vi "Object Tracking V2.vi"() -> ()   [LabVIEW 2019]
uses:
  <vilib>/userdefined/High Color/IMAQdx.ctl
  <vilib>/vision/Pattern Matching.llb/IMAQ Curve Parameters.ctl
  <vilib>/vision/driver/IMAQdx.llb/IMAQdx Buffer Number Mode.ctl
  <vilib>/vision/driver/NI_Vision_Acquisition_Software.lvlib
  <vilib>/vision/NI_Vision_Development_Module.lvlib
  <resource>/objmgr/imaqdx.rc
panel:
  out "Tracking":cluster{"x":dbl, "y":dbl}[](array[cluster])
  in  "Match Type":enum16{"Geometric Matching", "Pattern Matching"}(ring)=enum."Pattern Matching"
  in  "Match":bool
  out "Matches":T1(array[cluster]) {"Bounding Box"."y" format="%.2f"; "Bounding Box"."x" format="%.2f"; "Position"."y" format="%.2f"; "Position"."x" format="%.2f"; "Score" format="%.2f"; "Scale" format="%.2f"; "Angle" format="%.2f"}
  in  "Learn":bool
  in  "Snap Frame":bool
  in  "Camera Name":T2="cam0"
  in  "Stop Button":bool
  in  "Geometric Match Mode":T3={"Rotation"=TRUE, "Scale"=FALSE, "Occlusion"=FALSE, "Reserved"=FALSE, "Reserved"=FALSE, "Reserved"=FALSE}
  in  "Pattern Match Mode":u16(ring)=1 items=["Shift Invariant", "Rotation Invariant"]
  in  "Minimum Score":sgl=600.0
  in  "Nb of Matches":i32=1
  in  "Subpixel Accuracy":bool
  in  "Minimum Contrast":i32=10
  in  "Curve Parameters":T4={"Extraction Mode"=0, "Edge Threshold"=75, "Edge Filter Size"=1, "Min Length"=25, "Row Search Step Size"=15, "Col Search Step Size"=15, "Max Endpoint Gap"=10, "Closed"=FALSE, "Subpixel"=FALSE} {"Max Endpoint Gap" min=0; "Col Search Step Size" min=1 max=255 step=1; "Row Search Step Size" min=1 max=255 step=1; "Min Length" min=0; "Edge Filter Size" items=["Fine", "Normal", "Controur Tracing"]; "Edge Threshold" min=1 max=65535 step=1; "Extraction Mode" items=["Normal", "Uniform Regions"]}
  out "Template":T5(plugin-control)
  out "Snap Image":T5(plugin-control)
  out "Image Out":T5(plugin-control)
  # "1. Run the VI\n\n2. Click \"Snap Frame\" (make sure the object that you want to track\nit in the image at the time you snap the frame\n\n3. Use the mouse to select that object that you wish to track. This is done in the bottow left frame,\n\n4. Click \"Learn\" (This area is not saved at the new template image as seen in the bottom right frame)\n\n5. Click \"Match\" the program will then look for the template image and display the resutls with a red box."
  # "1."
  # "2."
  # "3."
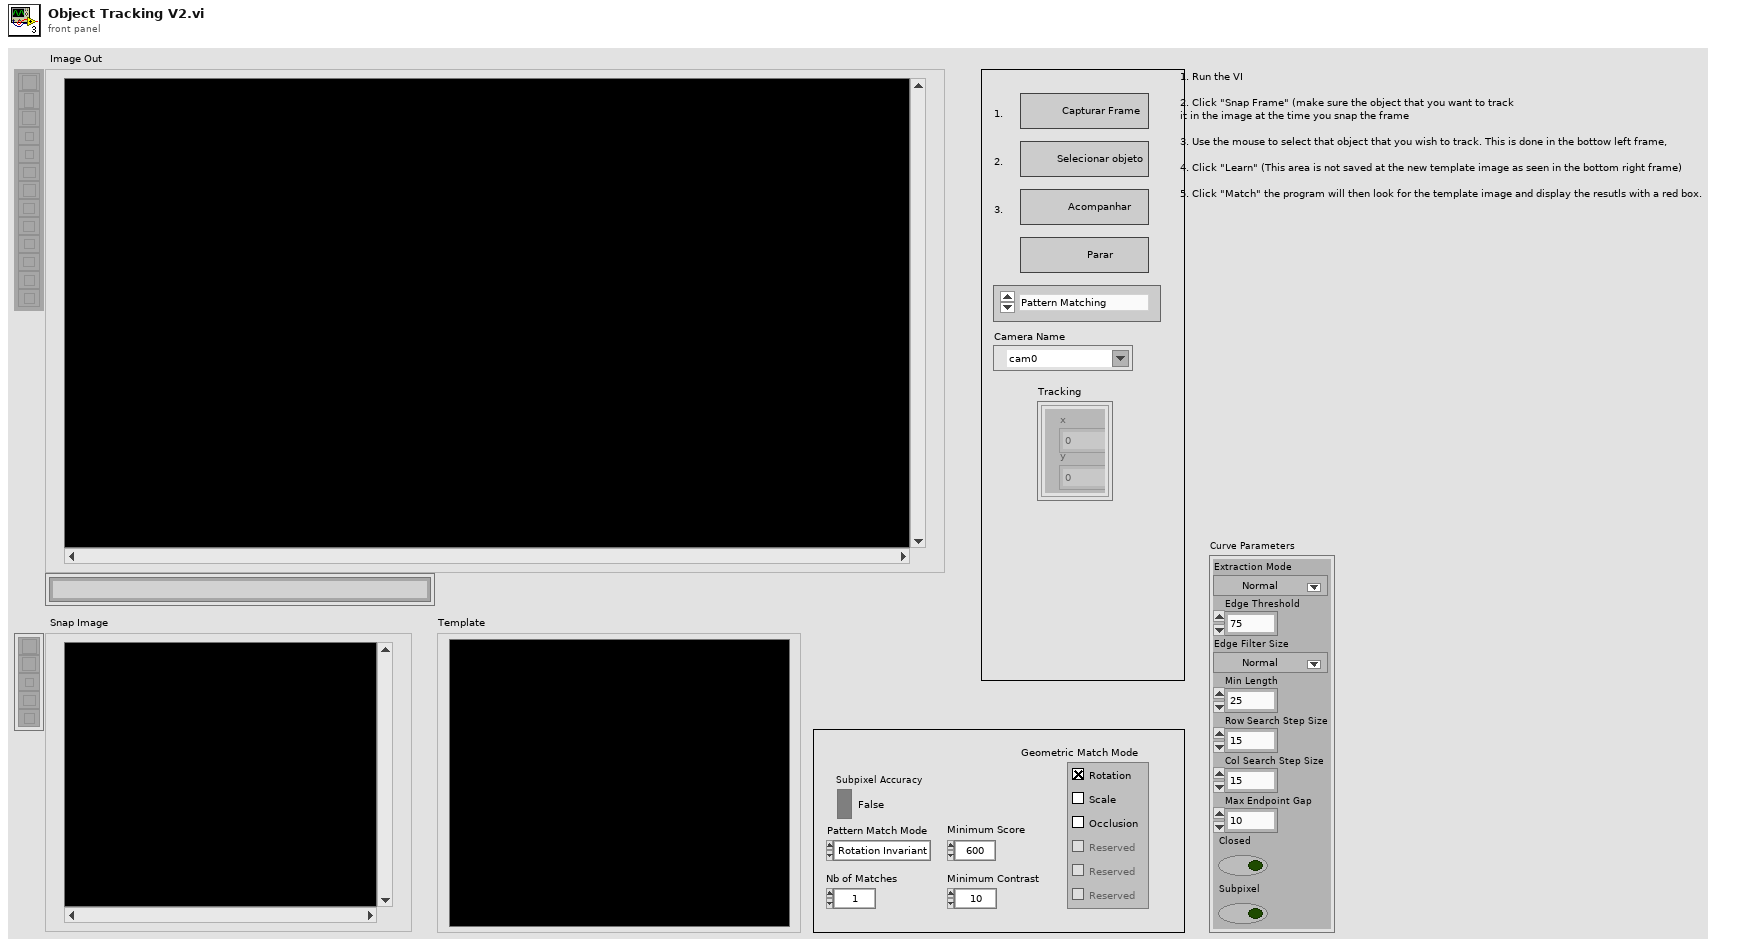
[diagram p1: front panel]
types:
  T1 = cluster{"Position":cluster{"x":sgl, "y":sgl}, "Angle":sgl, "Scale":sgl, "Score":sgl, "Bounding Box":cluster{"x":sgl, "y":sgl}[]}[]
  T2 = typedef "IMAQdx.ctl" = refnum<k21>
  T3 = cluster{"Rotation":bool, "Scale":bool, "Occlusion":bool, "Reserved":bool, "Reserved":bool, "Reserved":bool}
  T4 = typedef "IMAQ Curve Parameters.ctl" = cluster{"Extraction Mode":u32, "Edge Threshold":i32, "Edge Filter Size":u32, "Min Length":i32, "Row Search Step Size":i32, "Col Search Step Size":i32, "Max Endpoint Gap":i32, "Closed":bool, "Subpixel":bool}
  T5 = typedef "IMAQ Image.ctl" = refnum<image>
  T6 = cluster{"Global Rectangle":i32[], "Contours":cluster{"Contour Type":u32, "ROI Type":u32, "Points":i32[]}[]}
  T7 = typedef "NI_Vision_Acquisition_Software.lvlib/IMAQdx Buffer Number Mode.ctl" = enum32{"Next", "Last", "Buffer Number", "Every", "Last New"}
  T8 = cluster{i32[], cluster{"Contour Type":u32, "ROI Type":u32, i32[]}[]}
  T9 = typedef "Image Type" = u32
  T10 = typedef "IMAQ GM Match Report.ctl" = cluster{"Position":cluster{"x":sgl, "y":sgl}, "Angle":sgl, "Scale":sgl, "Score":sgl, "Bounding Box":cluster{"x":sgl, "y":sgl}[], "Contrast Reversed":bool, "Occlusion %":sgl, "Template Target Curve Score":sgl, "Target Template Curve Score":sgl, "Correlation Score":sgl}
  T11 = cluster{"Matches[0]":cluster{"Position":cluster{"x":sgl, "y":sgl}, "Angle":sgl, "Scale":sgl, "Score":sgl, "Bounding Box":cluster{"x":sgl, "y":sgl}[]}, "Matches[1]":cluster{"Position":cluster{"x":sgl, "y":sgl}, "Angle":sgl, "Scale":sgl, "Score":sgl, "Bounding Box":cluster{"x":sgl, "y":sgl}[]}, "Matches[2]":cluster{"Position":cluster{"x":sgl, "y":sgl}, "Angle":sgl, "Scale":sgl, "Score":sgl, "Bounding Box":cluster{"x":sgl, "y":sgl}[]}, "Matches[3]":cluster{"Position":cluster{"x":sgl, "y":sgl}, "Angle":sgl, "Scale":sgl, "Score":sgl, "Bounding Box":cluster{"x":sgl, "y":sgl}[]}, "Matches[4]":cluster{"Position":cluster{"x":sgl, "y":sgl}, "Angle":sgl, "Scale":sgl, "Score":sgl, "Bounding Box":cluster{"x":sgl, "y":sgl}[]}, "Matches[5]":cluster{"Position":cluster{"x":sgl, "y":sgl}, "Angle":sgl, "Scale":sgl, "Score":sgl, "Bounding Box":cluster{"x":sgl, "y":sgl}[]}, "Matches[6]":cluster{"Position":cluster{"x":sgl, "y":sgl}, "Angle":sgl, "Scale":sgl, "Score":sgl, "Bounding Box":cluster{"x":sgl, "y":sgl}[]}, "Matches[7]":cluster{"Position":cluster{"x":sgl, "y":sgl}, "Angle":sgl, "Scale":sgl, "Score":sgl, "Bounding Box":cluster{"x":sgl, "y":sgl}[]}, "Matches[8]":cluster{"Position":cluster{"x":sgl, "y":sgl}, "Angle":sgl, "Scale":sgl, "Score":sgl, "Bounding Box":cluster{"x":sgl, "y":sgl}[]}}
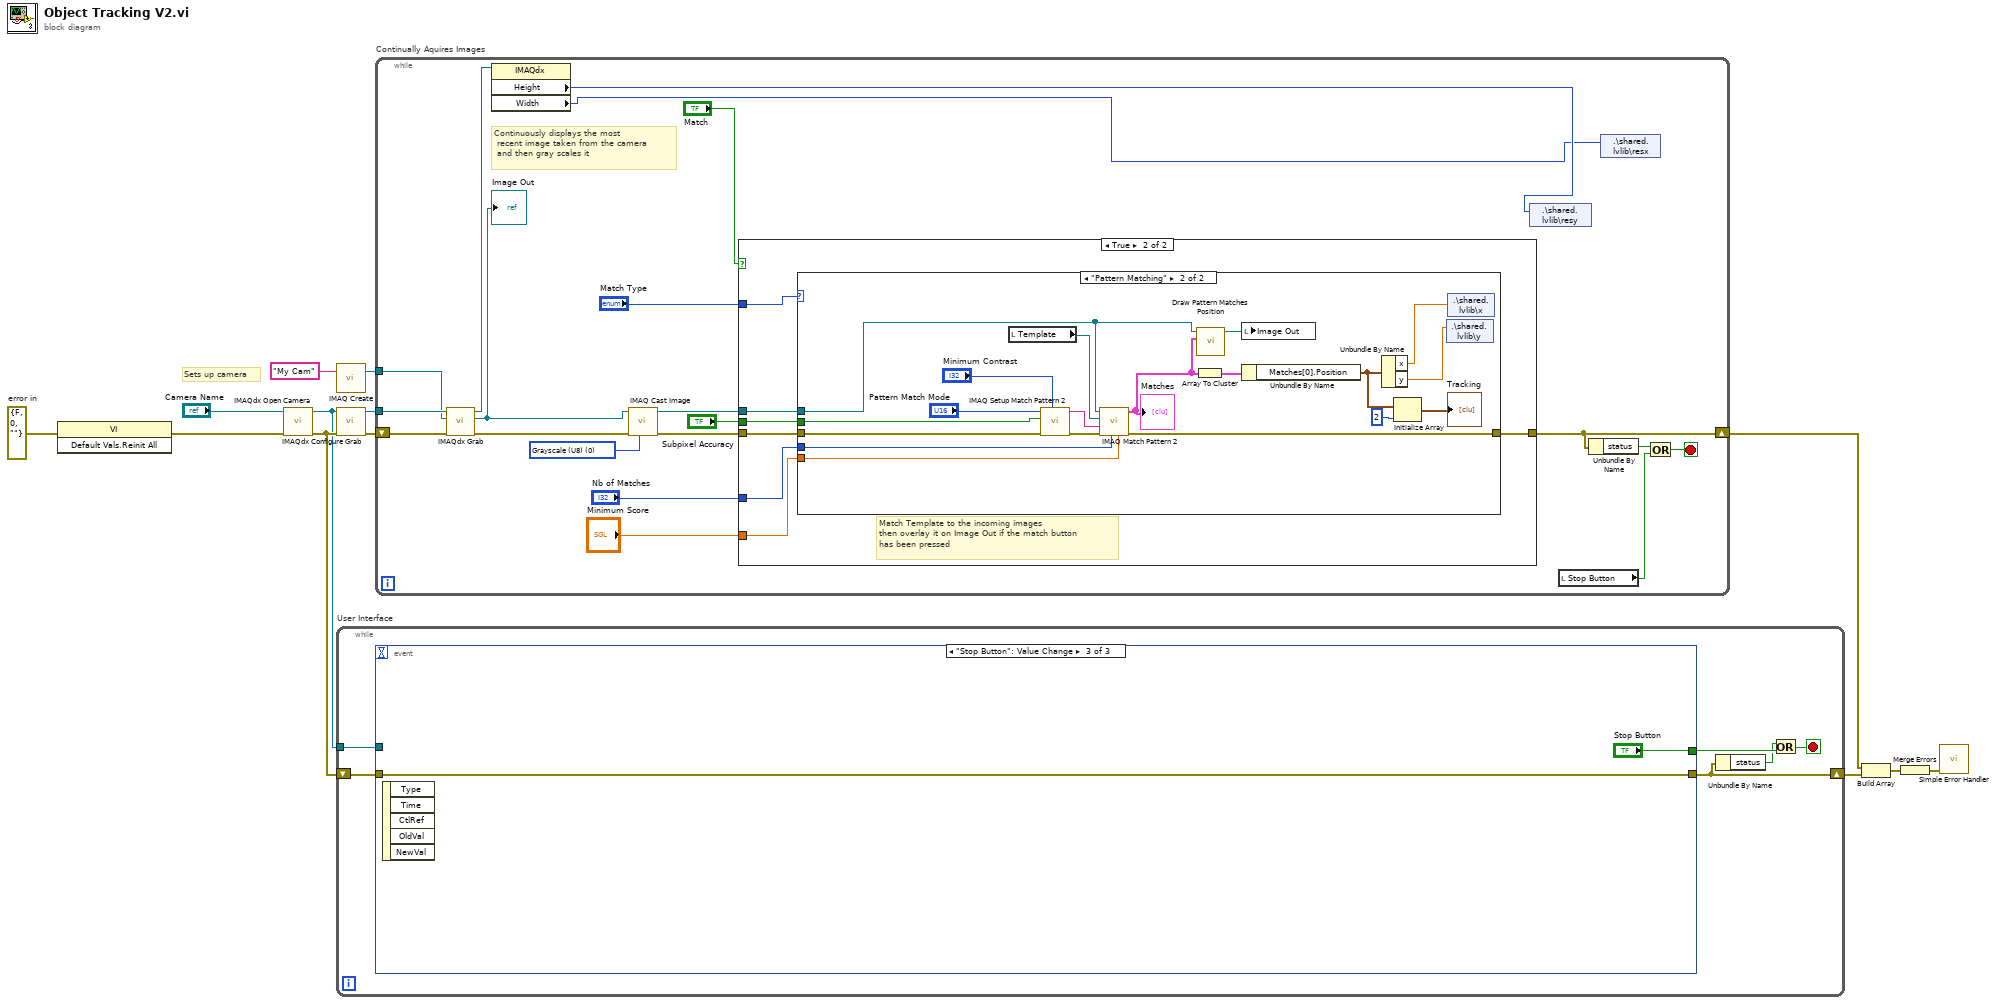
[diagram p0: block diagram]
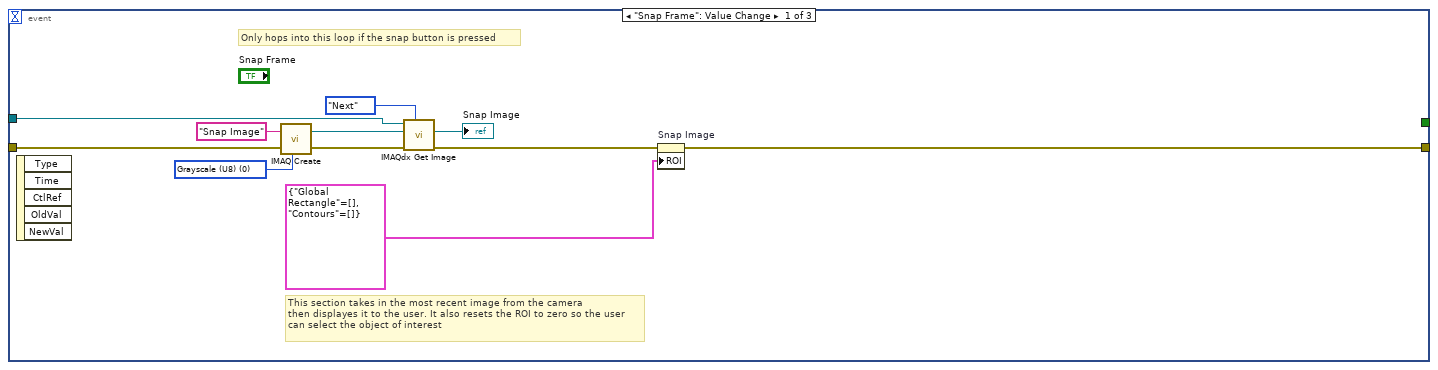
[diagram p2: hidden frame]
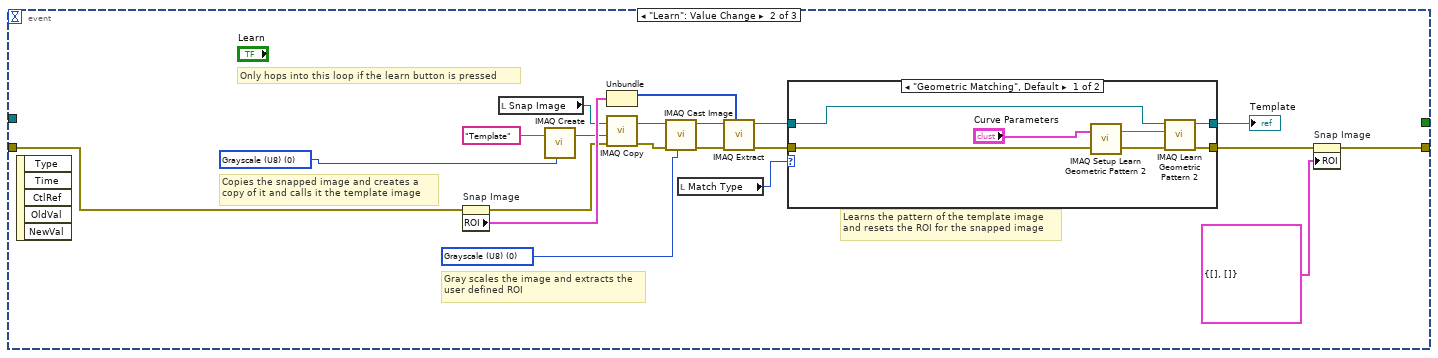
[diagram p3: hidden frame]
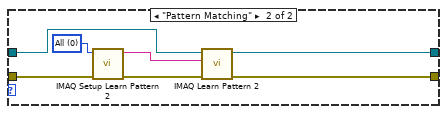
[diagram p4: hidden frame]
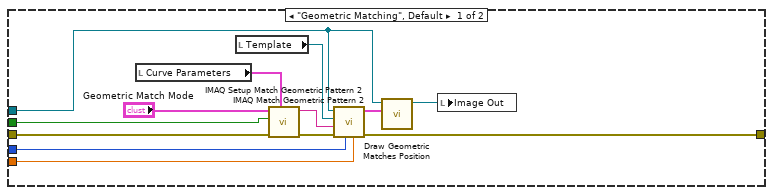
[diagram p6: hidden frame]
diagram:
  w10 = errorcluster {"status"=FALSE, "code"=0, "source"=""}  # error in
  # "Sets up camera"
  n1 = invoke class="VI" method="Default Vals.Reinit All"(error in=w10) -> (error out=w9:errorcluster)  [unwired: 2 in, 2 out]
  n2 = call <vilib>:"IMAQdx Open Camera.vi"("error in"=w9, "Session In"="Camera Name") -> ("error out"=w6:errorcluster, "Session Out"=w5:T2)  [unwired: 8 in]
  n3 = call "IMAQ Create"("Image Name"="My Cam") -> ("New Image"=w8:T5)  [unwired: 4 in, 1 out]
  n4 = call <vilib>:"IMAQdx Configure Grab.vi"("error in"=w6, "Session In"=w5) -> ("error out"=w12:errorcluster, "Session Out"=w13:T2)  [unwired: 8 in]
  n5 = while "User Interface" {
    tunnel: w5 -> [w18]
    shift-right: [w15] -> w2
    shift-left: w6 -> [w19]
    stop <- w17 stop-if-true
    n6 = event shown="[2] \"Stop Button\": Value Change" {
      selector: _ -> [_ _ _]
      dyn-events: _ -> [_ _ _]
      timeout: _ -> [_ _ _]
      tunnel: [_ _ "Stop Button"] -> w16
      tunnel: w19 -> [w25 w48 w65]
      tunnel: w18 -> [w24 _ _]
      tunnel: [w20 w44 w65] -> w15
      event "Snap Frame": Value Change {
        w23 = T9 0 items=["Grayscale (U8)", "Grayscale (I16)", "Grayscale (SGL)", "Complex (CSG)", "RGB (U32)", "HSL (U32)", "RGB (U64)", "Grayscale (U16)"] ("Image Type")
        # "Only hops into this loop if the snap button is pressed"
        # "This section takes in the most recent image from the camera \nthen displayes it to the user. It also resets the ROI to zero so the user\ncan select the object of interest"
        n7 = event-data() -> ()  [unwired: 1 in, 5 out]
        n8 = call "IMAQ Create"("Image Name"="Snap Image", "Image Type"=w23, "error in (no error)"=w25) -> ("New Image"=w28:T5, "error out"=w27:errorcluster)  [unwired: 2 in]
        n9 = call <vilib>:"IMAQdx Get Image.vi"("Buffer Number Mode (Next)"=IMAQdx_Buffer_Number_Mode."Next", "error in"=w27, "Image In"=w28, "Session In"=w24) -> ("error out"=w22:errorcluster, "Image Out"=→"Snap Image":T5)  [unwired: 4 in, 2 out]
        n10 = property on="Snap Image" class="ImageControl"(error in=w22, "ROI"=T6 {"Global Rectangle"=[], "Contours"=[]}) -> (error out=w20:errorcluster)  [unwired: 1 in, 1 out]
      }
      event "Learn": Value Change {
        w37 = T9 0 items=["Grayscale (U8)", "Grayscale (I16)", "Grayscale (SGL)", "Complex (CSG)", "RGB (U32)", "HSL (U32)", "RGB (U64)", "Grayscale (U16)"] ("Image Type")
        w38 = T9 0 items=["Grayscale (U8)", "Grayscale (I16)", "Grayscale (SGL)", "Complex (CSG)", "RGB (U32)", "HSL (U32)", "RGB (U64)", "Grayscale (U16)"] ("Image Type")
        # "Learns the pattern of the template image\nand resets the ROI for the snapped image"
        # "Gray scales the image and extracts the\nuser defined ROI"
        # "Copies the snapped image and creates a \ncopy of it and calls it the template image"
        # "Only hops into this loop if the learn button is pressed"
        n11 = event-data() -> ()  [unwired: 1 in, 5 out]
        n12 = property on="Snap Image" class="ImageControl"(error in=w48) -> (error out=w39:errorcluster, "ROI"=w47:T6)  [unwired: 1 in, 1 out]
        n13 = local read "Snap Image"() -> (w42:T5)
        n14 = call "IMAQ Create"("Image Name"="Template", "Image Type"=w38) -> ("New Image"=w41:T5)  [unwired: 3 in, 1 out]
        n15 = Unbundle(w47) -> ("Global Rectangle"=w46:i32[])  [unwired: 1 out]
        n16 = call "IMAQ Copy"("error in (no error)"=w39, "Image Dst"=w41, "Image Src"=w42) -> ("error out"=w34:errorcluster, "Image Dst Out"=w36:T5)  [unwired: 3 in]
        n17 = call "IMAQ Cast Image"("Image Type"=w37, "error in (no error)"=w34, "Image Src"=w36) -> ("error out"=w33:errorcluster, "Image Dst Out"=w35:T5)  [unwired: 7 in]
        n18 = local read "Match Type"() -> (w32:enum16{"Geometric Matching", "Pattern Matching"})
        n19 = call "IMAQ Extract"("Optional Rectangle"=w46, "error in (no error)"=w33, "Image Src"=w35) -> ("error out"=w31:errorcluster, "Image Dst Out"=w50:T5)  [unwired: 3 in, 4 out]
        n20 = case shown="\"Geometric Matching\", Default" w32 {
          tunnel: w50 -> [w53 w63]
          tunnel: [w54 w61] -> w49
          tunnel: [w55 w59] -> w45
          tunnel: w31 -> [w52 w58]
          frame "Geometric Matching", Default {
            n21 = call "IMAQ Setup Learn Geometric Pattern 2"("error in (no error)"=w52, "Curve Parameters"="Curve Parameters") -> ("error out"=w51:errorcluster, "Learn Geometric Pattern 2 Setup Data"=w56:string)
            n22 = call "IMAQ Learn Geometric Pattern 2"("error in (no error)"=w51, "Learn Geometric Pattern 2 Setup Data"=w56, "Template Image"=w53) -> ("error out"=w55:errorcluster, "Template Image Out"=w54:T5)  [unwired: 7 in]
          }
          frame "Pattern Matching" {
            w62 = u16 0 items=["All", "Shift Information", "Rotation Information"] ("Learn Mode")
            n23 = call "IMAQ Setup Learn Pattern 2"("error in (no error)"=w58, "Learn Mode"=w62) -> ("error out"=w60:errorcluster, "Learn Pattern Setup Data"=w64:string)  [unwired: 8 out]
            n24 = call "IMAQ Learn Pattern 2"("error in (no error)"=w60, "Learn Pattern Setup Data"=w64, "Image"=w63) -> ("error out"=w59:errorcluster, "Template Image Out"=w61:T5)  [unwired: 1 in, 6 out]
          }
        }
        "Template" <- w49
        n25 = property on="Snap Image" class="ImageControl"(error in=w45, "ROI"=T8 {[], []}) -> (error out=w44:errorcluster)  [unwired: 1 in, 1 out]
      }
      event "Stop Button": Value Change {
        n26 = event-data() -> ()  [unwired: 1 in, 5 out]
      }
    }
    n27 = Unbundle By Name(w15) -> ("status"=w14:bool)
    n28 = Or(x=w14, y=w16) -> (x .or. y?=w17:bool)
  }
  n29 = while "Continually Aquires Images" {
    tunnel: w13 -> [w86]
    tunnel: w8 -> [w84]
    shift-right: [w75] -> w3
    shift-left: w12 -> [w85]
    stop <- w76 stop-if-true
    w81 = T9 0 items=["Grayscale (U8)", "Grayscale (I16)", "Grayscale (SGL)", "Complex (CSG)", "RGB (U32)", "HSL (U32)", "RGB (U64)", "Grayscale (U16)"] ("Image Type")
    # "Continuously displays the most\n recent image taken from the camera\n and then gray scales it"
    n30 = call <vilib>:"IMAQdx Grab.vi"("error in"=w85, "Image In"=w84, "Session In"=w86) -> ("error out"=w82:errorcluster, "Image Out"=w83:T5, "Session Out"=w69:T2)  [unwired: 5 in, 1 out]
    "Image Out" <- w83
    n31 = property on="Property Node" class="IMAQdx"(reference=w69) -> ("Height"=w68:u32, "Width"=w67:u32)  [unwired: 1 in, 2 out]
    n32 = call "IMAQ Cast Image"("Image Type"=w81, "error in (no error)"=w82, "Image Src"=w83) -> ("error out"=w80:errorcluster, "Image Dst Out"=w79:T5)  [unwired: 7 in]
    n33 = case shown="True" "Match" {
      tunnel: w80 -> [w87 w94]
      tunnel: w79 -> [_ w93]
      tunnel: [w87 w92] -> w75
      tunnel: "Nb of Matches" -> [_ w91]
      tunnel: "Minimum Score" -> [_ w90]
      tunnel: "Subpixel Accuracy" -> [_ w89]
      tunnel: "Match Type" -> [_ w88]
      frame False {
      }
      frame True {
        # "Match Template to the incoming images \nthen overlay it on Image Out if the match button\nhas been pressed"
        n34 = case shown="\"Pattern Matching\"" w88 {
          tunnel: w94 -> [w100 w121]
          tunnel: w93 -> [w97 w116]
          tunnel: [w102 w120] -> w92
          tunnel: w91 -> [w99 w119]
          tunnel: w90 -> [w98 w118]
          tunnel: w89 -> [w96 w117]
          frame "Geometric Matching", Default {
            n35 = local read "Curve Parameters"() -> (w104:T4)
            n36 = local read "Template"() -> (w107:T5)
            n37 = call "IMAQ Setup Match Geometric Pattern 2"("Curve Parameters"=w104, "error in (no error)"=w100, "Subpixel Accuracy"=w96, "Match Mode"="Geometric Match Mode") -> ("error out"=w106:errorcluster, "Match Geometric Pattern 2 Setup Data"=w103:string)  [unwired: 6 in]
            n38 = call "IMAQ Match Geometric Pattern 2"("Minimum Match Score"=w98, "Number of Matches Requested"=w99, "error in (no error)"=w106, "Match Geometric Pattern 2 Setup Data"=w103, "Template Image"=w107, "Image"=w97) -> ("error out"=w102:errorcluster, "Matches (pixel)"=w95:T10[])  [unwired: 2 in, 2 out]
            n39 = call "Draw Geometric Matches Position .vi"("Matches (pixel)"=w95, "Image"=w97) -> ("Image Out"=w101:T5)  [unwired: 9 out]
            n40 = local write "Image Out"(w101) -> ()
          }
          frame "Pattern Matching" {
            n41 = local read "Template"() -> (w123:T5)
            n42 = call "IMAQ Setup Match Pattern 2"("Minimum Contrast"="Minimum Contrast", "error in (no error)"=w121, "Subpixel Accuracy"=w117, "Match Mode"="Pattern Match Mode") -> ("error out"=w122:errorcluster, "Match Pattern Setup Data"=w126:string)  [unwired: 1 in, 5 out]
            n43 = call "IMAQ Match Pattern 2"("Minimum Match Score"=w118, "Number of Matches Requested"=w119, "error in (no error)"=w122, "Match Pattern Setup Data"=w126, "Template Image"=w123, "Image"=w116) -> ("error out"=w120:errorcluster, "Matches"=w114:T1)  [unwired: 1 in, 3 out]
            "Matches" <- w114
            n44 = Array To Cluster(array=w114) -> (cluster=w113:T11)
            n45 = call "Draw Pattern Matches Position .vi"("Matches"=w114, "Image"=w116) -> ("Image Out"=w115:T5)  [unwired: 9 in]
            n46 = local write "Image Out"(w115) -> ()
            n47 = Unbundle By Name(w113) -> ("Matches[0].Position"=w111:cluster{"x":sgl, "y":sgl})
            n48 = Unbundle By Name(w111) -> ("x"=w109:sgl, "y"=w108:sgl)
            n49 = Initialize Array(w111, 2) -> (→"Tracking":cluster{"x":sgl, "y":sgl}[])
            n50 = shared-variable ".\\shared.lvlib\\y"(w108) -> ()  [unwired: 1 in, 1 out]
            n51 = shared-variable ".\\shared.lvlib\\x"(w109) -> ()  [unwired: 1 in, 1 out]
          }
        }
      }
    }
    n52 = shared-variable ".\\shared.lvlib\\resy"(w68) -> ()  [unwired: 1 in, 1 out]
    n53 = local read "Stop Button"() -> (w77:bool)
    n54 = Unbundle By Name(w75) -> ("status"=w74:bool)
    n55 = shared-variable ".\\shared.lvlib\\resx"(w67) -> ()  [unwired: 1 in, 1 out]
    n56 = Or(x=w74, y=w77) -> (x .or. y?=w76:bool)
  }
  n57 = Build Array(w3, w2) -> (w1:errorcluster[])
  n58 = Merge Errors(w1) -> (w4:errorcluster)
  n59 = call <vilib>:"Simple Error Handler.vi"("error in (no error)"=w4) -> ()  [unwired: 4 in, 5 out]
